vi "TV.vi"() -> ()   [LabVIEW 2018]
panel:
  in  "Threshold":sgl=0.075
  in  "Deblurr Image":bool
  in  "stop":bool
  in  "Kernel Angle":dbl
  in  "Kernel Radius":dbl=9.0
  in  "Kernel Length":dbl
  in  "Blur Type":enum32{"Radio Selection 1", "Radio Selection 2"}(radio)
  in  "Color":enum32{"Radio Selection 1", "Radio Selection 2"}(radio)=enum."Radio Selection 2"
  in  "Path":path=path "C:/Users/burro/Desktop/Demos/samford_OOF_blured.jpg"
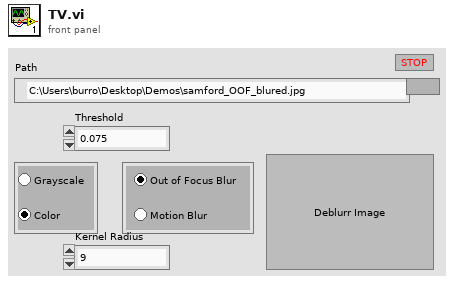
[diagram p1: front panel]
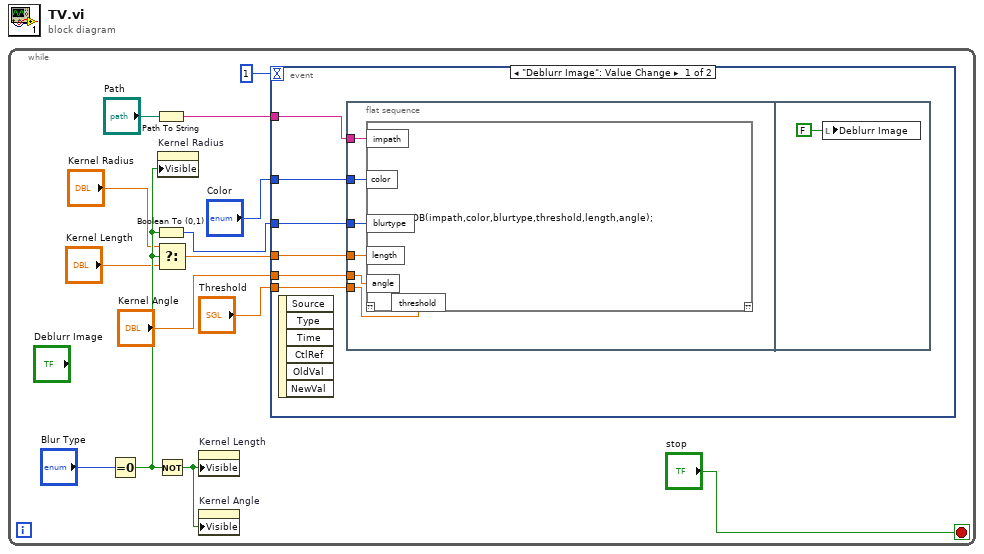
[diagram p0: block diagram]
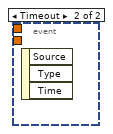
[diagram p2: hidden frame]
diagram:
  n1 = while {
    stop <- "stop" stop-if-true
    n2 = Equal To 0?(x="Blur Type") -> (x = 0?=w5:bool)
    n3 = Path To String(path="Path") -> (string=w7:string)
    n4 = Boolean To (0,1)(Boolean=w5) -> (0, 1=w14:i16)
    n5 = Select(t="Kernel Radius", s=w5, f="Kernel Length") -> (s? t:f=w13:dbl)
    n6 = Not(x=w5) -> (.not. x?=w11:bool)
    n7 = property on="Kernel Radius" class="DigNum (strict)"("Visible"=w5) -> ()  [unwired: 2 in, 2 out]
    n8 = property on="Kernel Length" class="DigNum (strict)"("Visible"=w11) -> ()  [unwired: 2 in, 2 out]
    n9 = property on="Kernel Angle" class="DigNum (strict)"("Visible"=w11) -> ()  [unwired: 2 in, 2 out]
    n10 = event shown="[0] \"Deblurr Image\": Value Change" {
      selector: _ -> [_ _]
      dyn-events: _ -> [_ _]
      timeout: 1 -> [_ _]
      tunnel: w7 -> [w20 _]
      tunnel: "Color" -> [w19 _]
      tunnel: w14 -> [w18 _]
      tunnel: w13 -> [w17 _]
      tunnel: "Kernel Angle" -> [w16 _]
      tunnel: "Threshold" -> [w15 _]
      event "Deblurr Image": Value Change {
        n11 = event-data() -> ()  [unwired: 1 in, 6 out]
        n12 = flat-sequence {
          tunnel: w15 -> [w21]
          tunnel: w20 -> [w22]
          tunnel: w19 -> [w26]
          tunnel: w18 -> [w25]
          tunnel: w17 -> [w24]
          tunnel: w16 -> [w23]
          frame #0 {
            n13 = script code="LVMLTVDB(impath,color,blurtype,threshold,length,angle);"("color"=w26, "blurtype"=w25, "length"=w24, "angle"=w23, "impath"=w22, "threshold"=w21) -> ()  [unwired: 1 in, 1 out]
          }
          frame #1 {
            n14 = local write "Deblurr Image"(FALSE ("Deblurr Image")) -> ()
          }
        }
      }
      event Timeout {
        n15 = event-data() -> ()  [unwired: 1 in, 3 out]
      }
    }
  }
